vi "getFillPositionNumbers.vi"(8 "error in (no error)":errorcluster, 10 "Array":i32[](array[numeric]), 11 "DIO64Output in":refnum<class "DIO64Output.lvclass">) -> (0 "error out":errorcluster, 1 "fill number":i32[](array[numeric]), 2 "position":i32[](array[numeric]), 3 "DIO64Output out":refnum<class "DIO64Output.lvclass">)   [LabVIEW 2009, in "Hardware.lvlib" / "Channels.lvlib" / "DIO64Output.lvclass"]
uses:
  DIO64Output.lvclass
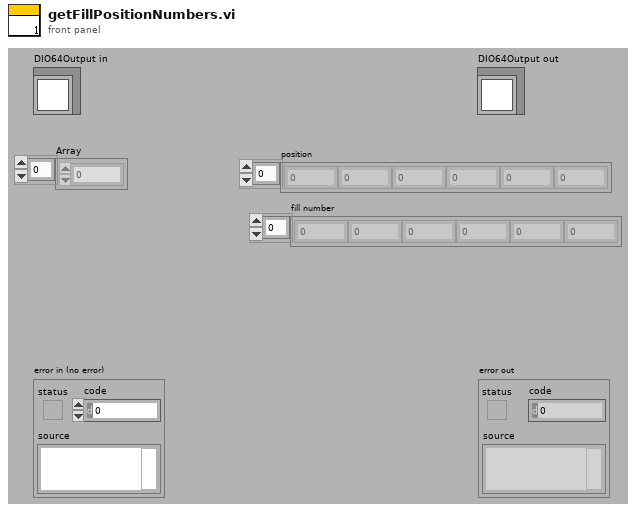
[diagram p1: front panel]
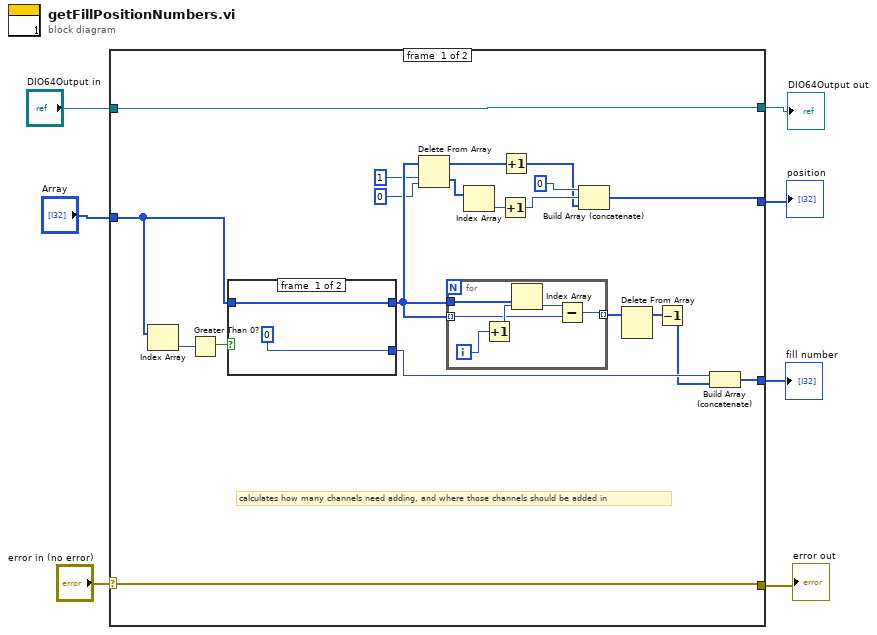
[diagram p0: block diagram]
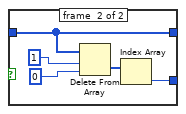
[diagram p2: hidden frame]
diagram:
  n1 = case shown="No Error" "error in (no error)" {
    selector: "error in (no error)" -> [w26 w42]
    tunnel: [w26 w42] -> w6
    tunnel: [w27 w41] -> w4
    tunnel: "DIO64Output in" -> [w27 w41]
    tunnel: "Array" -> [w10 _]
    tunnel: [w9 _] -> w1
    tunnel: [w8 _] -> w2
    frame #0 {
      # "calculates how many channels need adding, and where those channels should be added in"
      n2 = Index Array(array=w10) -> (element=w25:i32)  [unwired: 1 in]
      n3 = Greater Than 0?(x=w25) -> (x > 0?=w24:bool)
      n4 = case shown="True" w24 {
        tunnel: w10 -> [w35 w36]
        tunnel: [w35 w36] -> w20
        tunnel: [0 w38] -> w22
        frame #0 {
        }
        frame #1 {
          n5 = Delete From Array(array=w36, length=1, index=0) -> (deleted portion=w37:i32[])  [unwired: 1 out]
          n6 = Index Array(array=w37) -> (element=w38:i32)  [unwired: 1 in]
        }
      }
      n7 = Delete From Array(array=w20, length=1, index=0) -> (deleted portion=w17:i32[], array with subset deleted=w12:i32[])
      n8 = for {
        tunnel: w20 -> [w33]
        tunnel: w20 -> [w29] mode=indexing
        tunnel: [w28] -> w23 mode=indexing
        i -> [w31]
        n9 = Increment(x=w31) -> (x+1=w32:i32)
        n10 = Index Array(array=w33, index=w32) -> (element=w30:i32)
        n11 = Subtract(x=w30, y=w29) -> (x-y=w28:i32)
      }
      n12 = Index Array(array=w17) -> (element=w15:i32)  [unwired: 1 in]
      n13 = Increment(x=w15) -> (x+1=w13:i32)
      n14 = Increment(x=w12) -> (x+1=w11:i32[])
      n15 = Build Array (concatenate)(0, w13, w11) -> (w9:i32[])
      n16 = Delete From Array(array=w23) -> (array with subset deleted=w21:i32[])  [unwired: 2 in, 1 out]
      n17 = Decrement(x=w21) -> (x-1=w16:i32[])
      n18 = Build Array (concatenate)(w22, w16) -> (w8:i32[])
    }
    frame #1 {
    }
  }
  "error out" <- w6
  "DIO64Output out" <- w4
  "fill number" <- w2
  "position" <- w1
